vi "Set time.vi"(7 "[x]":T1, 8 "error in (no error)":errorcluster, 10 "Time (array)":dbl[](array[numeric]), 11 "Serial Port in":refnum<visa-resource-name>) -> (0 "error out":errorcluster, 3 "Serial Port out":refnum<visa-resource-name>)   [LabVIEW 2016, in "Chemyx_Syringe_Pump_driver.lvlib"]
doc: "Sets the times of the syringe multiple-step operations.\n\nTime is an array of double floats. Units are hours."
uses:
  Chemyx_Syringe_Pump_driver.lvlib
  _private/Control/Control Mode.ctl
panel:
  # "Sets the times of the syringe operations"
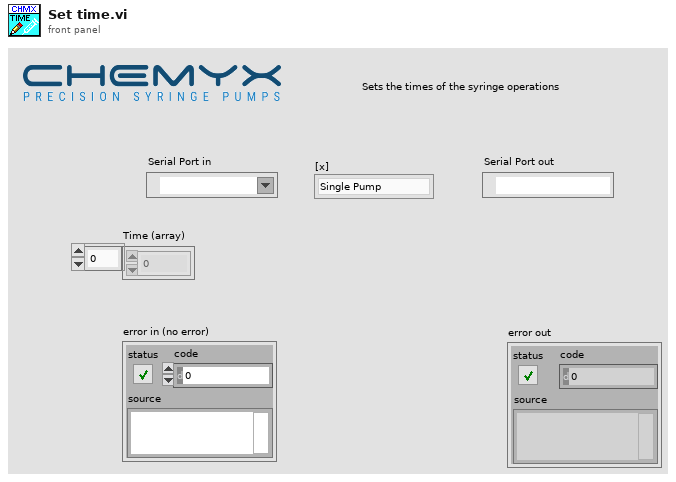
[diagram p1: front panel]
types:
  T1 = typedef "Chemyx_Syringe_Pump_driver.lvlib/Control Mode.ctl" = enum16{"Single Pump", "Pump Chanel 1", "Pump Channel 2", "Cycle Mode"}
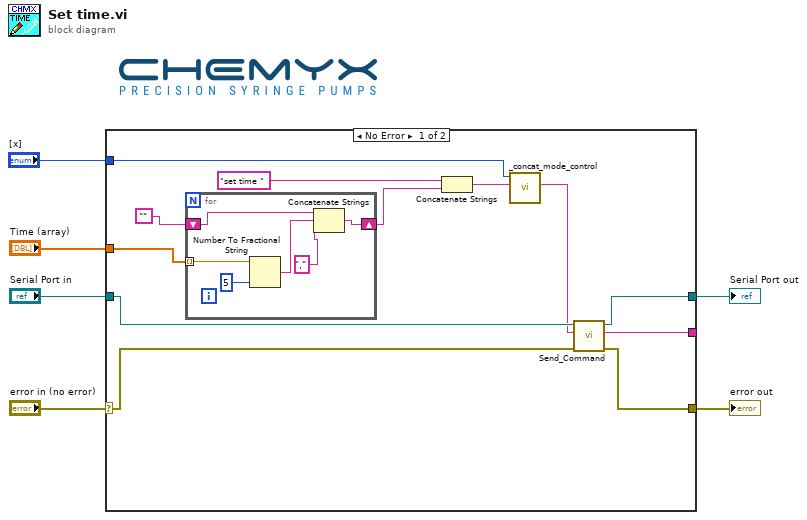
[diagram p0: block diagram]
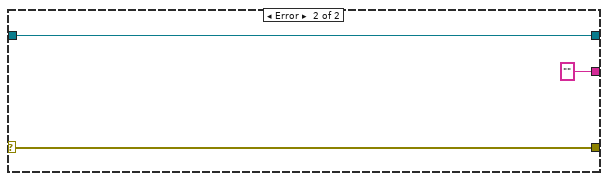
[diagram p2: hidden frame]
diagram:
  n1 = case shown="No Error" "error in (no error)" {
    selector: "error in (no error)" -> [w17 w27]
    tunnel: "Serial Port in" -> [w18 w26]
    tunnel: [w16 w27] -> w4
    tunnel: [w15 w26] -> w3
    tunnel: "Time (array)" -> [w13 _]
    tunnel: [w12 "" ("Read buffer")] -> _
    tunnel: "[x]" -> [w7 _]
    frame No Error {
      n2 = for {
        tunnel: w13 -> [w20] mode=indexing
        shift-right: [w24] -> w10
        shift-left: "" -> [w23]
        n3 = Number To Fractional String(number=w20, precision (6)=i16 5) -> (F-format string=w22:string)  [unwired: 2 in]
        n4 = Concatenate Strings(w23, w22, ",") -> (w24:string)
      }
      n5 = Concatenate Strings("set time ", w10) -> (w9:string)
      n6 = call "_concat_mode_control.vi"("write buffer"=w9, "[x]"=w7) -> ("write buffer out"=w8:string)  [unwired: 9 in]
      n7 = call "Send_Command.vi"("error in (no error)"=w17, "write buffer"=w8, "Serial Port in"=w18) -> ("error out"=w16:errorcluster, "Read buffer"=w12:string, "VISA Refnum out"=w15:refnum<visa-resource-name>)  [unwired: 6 in]
    }
    frame Error {
    }
  }
  "error out" <- w4
  "Serial Port out" <- w3
